vi "Userdefined Symbol AE.vi"(8 "错误输入":errorcluster, 10 "Index":i32, 11 "Listbox Ref":refnum<vi>) -> (0 "错误输出":errorcluster, 2 "Image":T1 caption="图像", 3 "Dup Listbox Ref":refnum<vi>)   [LabVIEW 2012, in "Listbox Tool.lvlib"]
uses:
  Listbox Tool.lvlib
  <vilib>/picture/picture.llb/imagedata.ctl
panel:
  in  "图像":T1
  in  "Mode":enum16{"Set", "Get", "Restore"}(ring)
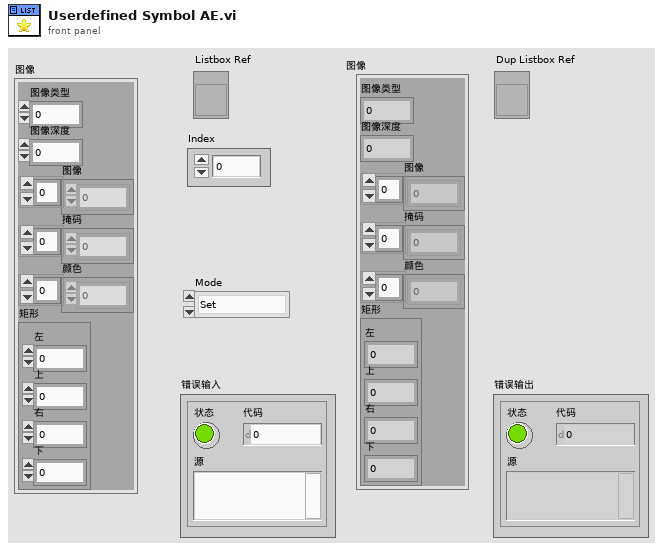
[diagram p1: front panel]
types:
  T1 = typedef "imagedata.ctl" = cluster{"image type":i32, "image depth":i32, "image":u8[], "mask":u8[], "colors":u32[], "Rectangle":cluster{"left":i16, "top":i16, "right":i16, "bottom":i16}}
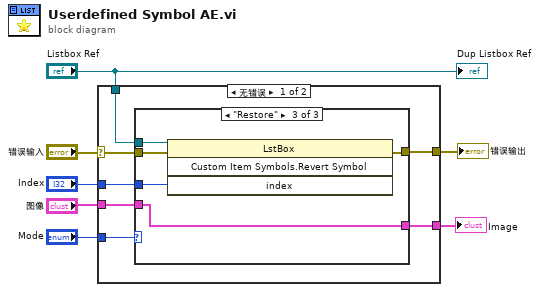
[diagram p0: block diagram]
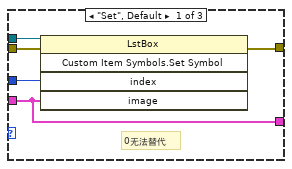
[diagram p2: hidden frame]
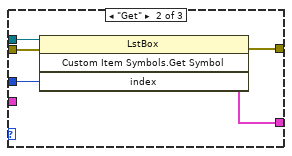
[diagram p3: hidden frame]
diagram:
  n1 = case shown="无错误" "错误输入" {
    selector: "错误输入" -> [w13 w30]
    tunnel: [w12 w30] -> w6
    tunnel: "Listbox Ref" -> [w14 _]
    tunnel: "Index" -> [w11 _]
    tunnel: [w10 _] -> w3
    tunnel: "Mode" -> [w9 _]
    tunnel: "图像" -> [w8 _]
    frame No Error {
      n2 = case shown="\"Restore\"" w9 {
        tunnel: w14 -> [w18 w24 w28]
        tunnel: w13 -> [w19 w23 w29]
        tunnel: [w17 w22 w27] -> w12
        tunnel: w11 -> [w16 w21 w25]
        tunnel: [w15 w20 w26] -> w10
        tunnel: w8 -> [w15 _ w26]
        frame "Set", Default {
          # "0无法替代"
          n3 = invoke class="LstBox" method="Custom Item Symbols.Set Symbol"(reference=w18, error in=w19, "index"=w16, "image"=w15) -> (error out=w17:errorcluster)  [unwired: 1 in, 4 out]
        }
        frame "Get" {
          n4 = invoke class="LstBox" method="Custom Item Symbols.Get Symbol"(reference=w24, error in=w23, "index"=w21) -> (error out=w22:errorcluster, "Custom Item Symbols:Get Symbol"=w20:T1)  [unwired: 1 in, 2 out]
        }
        frame "Restore" {
          n5 = invoke class="LstBox" method="Custom Item Symbols.Revert Symbol"(reference=w28, error in=w29, "index"=w25) -> (error out=w27:errorcluster)  [unwired: 1 in, 3 out]
        }
      }
    }
    frame Error {
    }
  }
  "错误输出" <- w6
  "Image" <- w3
  "Dup Listbox Ref" <- "Listbox Ref"
